vi "Global 1.vi"() -> ()   [LabVIEW 2016]
panel:
  in  "Positions":dbl
  in  "Distance":dbl=129.9598
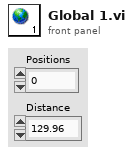
[diagram p1: front panel]
diagram:
